vi "LimitationIfNotNaN.vi"(8 "x":dbl format="%#_13g", 10 "Minimal Power":dbl=nan, 11 "Maximum Power":dbl=nan) -> (2 "In Range?":bool, 3 "Power Out":dbl)   [LabVIEW 2017]
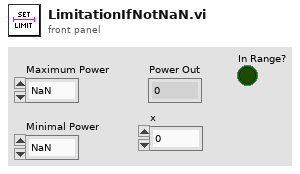
[diagram p1: front panel]
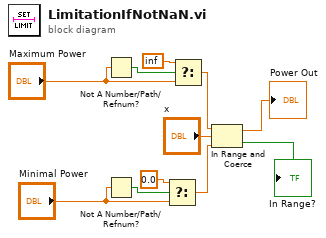
[diagram p0: block diagram]
diagram:
  n1 = Not A Number/Path/Refnum?(number/path/refnum="Maximum Power") -> (NaN/Path/Refnum?=w4:bool)
  n2 = Not A Number/Path/Refnum?(number/path/refnum="Minimal Power") -> (NaN/Path/Refnum?=w5:bool)
  n3 = Select(t=0.0, s=w5, f="Minimal Power") -> (s? t:f=w7:dbl)
  n4 = Select(t=inf, s=w4, f="Maximum Power") -> (s? t:f=w8:dbl)
  n5 = In Range and Coerce(upper limit=w8, x="x", lower limit=w7) -> (coerced(x)=→"Power Out":dbl, In Range?=→"In Range?":bool)
